vi "writeToXML.vi"(8 "error in (no error)":errorcluster, 10 "ClassLabel":string, 11 "FixedTarget in":refnum<class "FixedTarget.lvclass">) -> (0 "error out":errorcluster, 2 "XMLout":string, 3 "FixedTarget out":refnum<class "FixedTarget.lvclass">)   [LabVIEW 2022 SP3, in "TCSDataDefinitions.lvlib" / "TCSCommand.lvlib" / "TargetConfiguration.lvlib" / "Target.lvlib" / "FixedTarget.lvlib" / "FixedTarget.lvclass"]
uses:
  FixedTarget.lvclass
  <userlib>/Common/UnitsAndXML/FlattenItemWithUnitToXML/FlattenPlaneAngleToXML/PlaneAngleUnit.ctl
  <userlib>/Common/UnitsAndXML/FlattenItemWithUnitToXML/FlattenVelocityToXML/VelocityUnit.ctl
  FixedTarget.lvclass/FixedTarget.ctl
  Target/Target.lvclass
  ProperMotion/ProperMotion.lvclass
  <userlib>/Common/UnitsAndXML/UnitsAndXML.lvlib
  <userlib>/Common/XML/XMLGenerator/XMLGenerator.lvclass
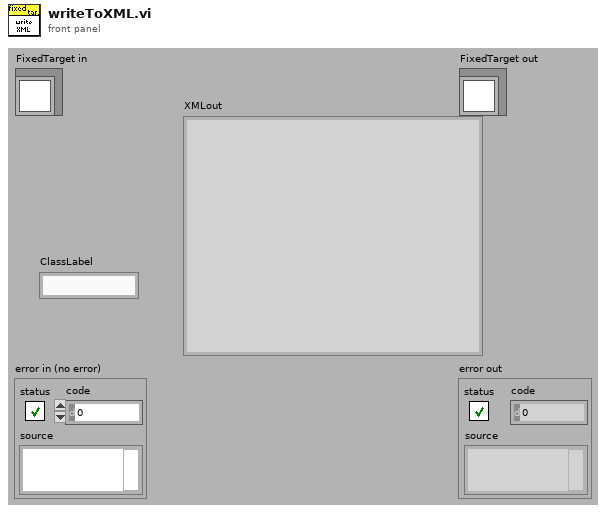
[diagram p1: front panel]
types:
  T1 = typedef "UnitsAndXML.lvlib/VelocityUnit.ctl" = enum16{"m/s", "km/s", "kn"}
  T2 = typedef "UnitsAndXML.lvlib/PlaneAngleUnit.ctl" = enum16{"rad", "deg", "'", "\""}
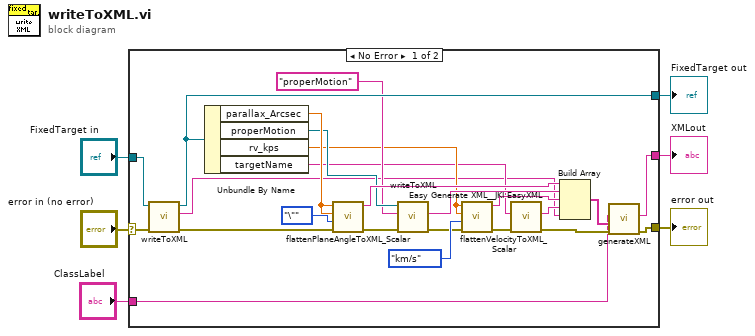
[diagram p0: block diagram]
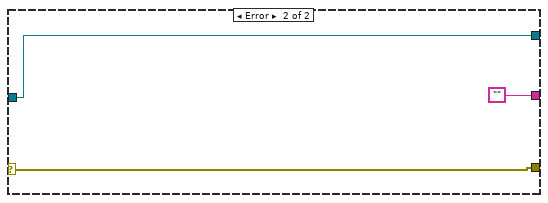
[diagram p2: hidden frame]
diagram:
  n1 = case shown="No Error" "error in (no error)" {
    selector: "error in (no error)" -> [w28 w33]
    tunnel: [w12 w33] -> w5
    tunnel: [w29 w32] -> w3
    tunnel: "FixedTarget in" -> [w30 w32]
    tunnel: "ClassLabel" -> [w7 _]
    tunnel: [w9 ""] -> w1
    frame No Error {
      n2 = call-parent "writeToXML.vi"("error in (no error)"=w28, "Target in"=w30) -> ("error out"=w25:errorcluster, "XML out"=w8:string, "Target out"=w29:refnum<class "FixedTarget.lvclass">)  [unwired: 7 in]
      n3 = Unbundle By Name(w29) -> ("parallax_Arcsec"=w27:dbl[unit], "properMotion"=w23:refnum<class "ProperMotion.lvclass">, "rv_kps"=w19:dbl[unit], "targetName"=w15:string)
      n4 = call <userlib>:"flattenPlaneAngleToXML_Scalar.vi"("error in (no error)"=w25, "planeAngleUnitInXML"=PlaneAngleUnit."\"", "planeAngleAgain"=w27, "planeAngle"=w27) -> ("error out"=w20:errorcluster, "xmlString"=w24:string)  [unwired: 6 in]
      n5 = call-dynamic "writeToXML.vi"("error in (no error)"=w20, "ClassLabel"="properMotion", "ProperMotion in"=w23) -> ("error out"=w17:errorcluster, "XMLout"=w21:string)  [unwired: 6 in, 1 out]
      n6 = call <userlib>:"flattenVelocityToXML_Scalar.vi"("error in (no error)"=w17, "velocityUnitInXML"=VelocityUnit."km/s", "velocityAgain"=w19, "velocity"=w19) -> ("error out"=w14:errorcluster, "xmlString"=w16:string)  [unwired: 6 in]
      n7 = call <vilib>:"Easy Generate XML__JKI EasyXML.vi"("error in (no error)"=w14, "LabVIEW Data"=w15) -> ("error out"=w13:errorcluster, "XML String"=w11:string)  [unwired: 8 in]
      n8 = Build Array(w24, w21, w16, w11, w8) -> (w10:string[])
      n9 = call <userlib>:"generateXML.vi"("error in"=w13, "childrenXML"=w10, "elementName"=w7) -> ("error out"=w12:errorcluster, "XML out"=w9:string)  [unwired: 6 in, 1 out]
    }
    frame Error {
    }
  }
  "error out" <- w5
  "FixedTarget out" <- w3
  "XMLout" <- w1
